vi "XML Add Valves.vi"() -> ()   [LabVIEW 2011]
panel:
  in  "XML Output":string
  in  "XML Input":string
  in  "Valves":T1(array[cluster])
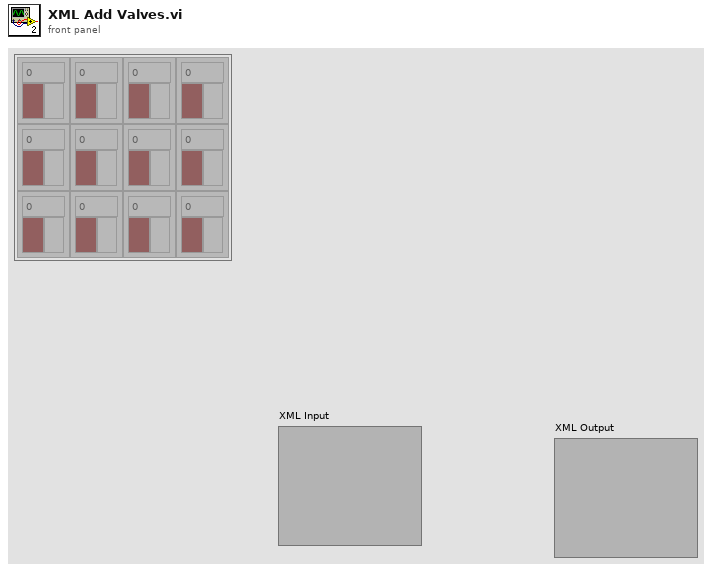
[diagram p1: front panel]
types:
  T1 = cluster{"Index":dbl, "Enabled":bool, "Value":bool}[][]
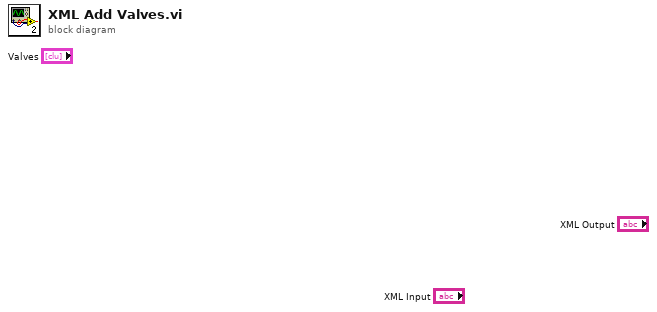
[diagram p0: block diagram]
diagram:
